vi "RiferimentoTensioneKEB.vi"(11 "Value in":cluster{"Hz":dbl, "V":dbl}) -> (3 "Riferimento Tensione":sgl)   [LabVIEW 2019]
uses:
  Global config keb.vi
  KEB VF status global.vi
panel:
  out "correzione V %":dbl
  in  "%":dbl format="%#_13g"
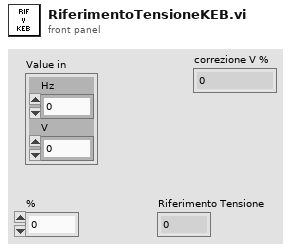
[diagram p1: front panel]
types:
  T1 = typedef "ConfigurazioneKeb.ctl" = cluster{"Freq nom":dbl, "RPM nom":dbl, "Pot nom":dbl, "I nom":dbl, "V nom":dbl, "Rpm max":dbl, "Tipo Motore":dbl}
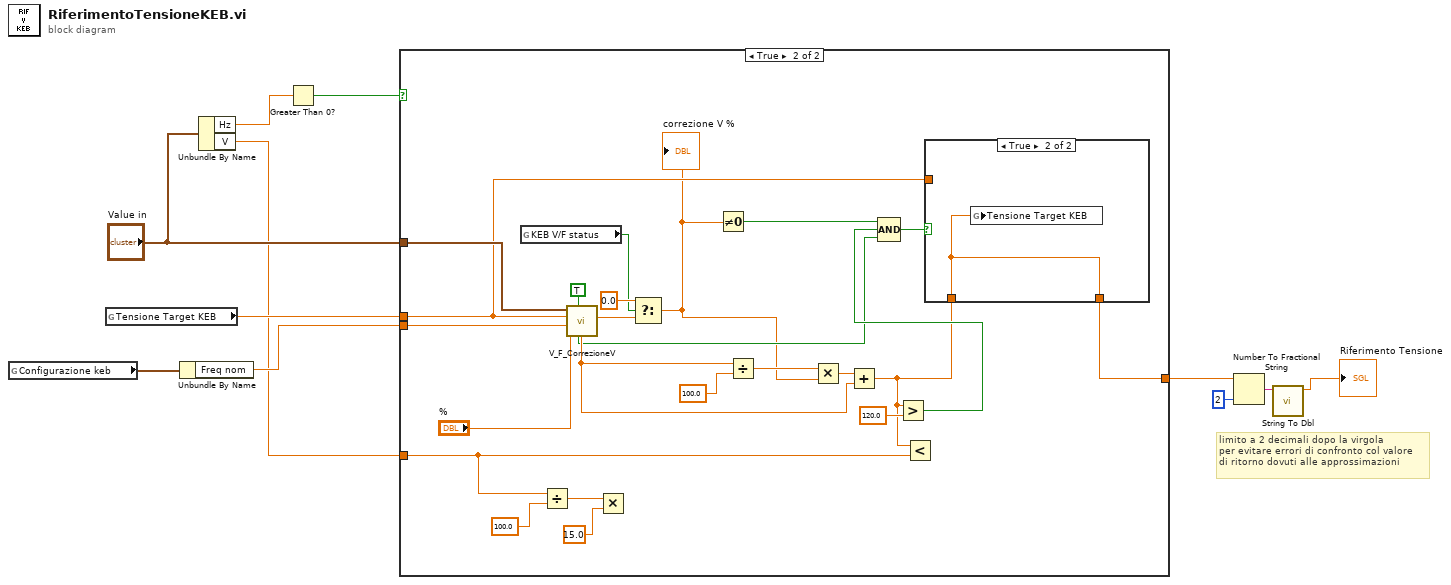
[diagram p0: block diagram]
diagram:
  # "limito a 2 decimali dopo la virgola\nper evitare errori di confronto col valore\ndi ritorno dovuti alle approssimazioni"
  n1 = global read "Global config keb.vi" "Configurazione keb"() -> (w11:T1)
  n2 = global read "Global config keb.vi" "Tensione Target KEB"() -> (w9:dbl)
  n3 = Unbundle By Name(w11) -> ("Freq nom"=w10:dbl)
  n4 = Unbundle By Name("Value in") -> ("Hz"=w7:dbl, "V"=w6:dbl)
  n5 = Greater Than 0?(x=w7) -> (x > 0?=w5:bool)
  n6 = case shown="True" w5 {
    tunnel: w10 -> [_ w33]
    tunnel: "Value in" -> [_ w32]
    tunnel: w9 -> [w12 w23]
    tunnel: [w12 w24] -> w2
    tunnel: w6 -> [_ w17]
    frame False {
    }
    frame True {
      n7 = global read "KEB VF status global.vi" "KEB V/F status"() -> (w13:bool)
      n8 = Divide(x=w17, y=100.0) -> (x/y=w20:dbl)
      n9 = call "V_F_CorrezioneV.vi"("Limita"=TRUE, "%"="%", "Fginocchio"=w33, "Vmax"=w23, "Value in"=w32) -> ("correzione V %"=w16:dbl, "In Range?"=w18:bool)  [unwired: 1 in, 4 out]
      n10 = Multiply(x=w20, y=15.0) -> ()  [unwired: 1 out]
      n11 = Select(t=0.0, s=w13, f=w16) -> (s? t:f=w14:dbl)
      "correzione V %" <- w14
      n12 = Not Equal To 0?(x=w14) -> (x != 0?=w27:bool)
      n13 = Divide(x=w23, y=100.0) -> (x/y=w30:dbl)
      n14 = Multiply(x=w30, y=w14) -> (x*y=w29:dbl)
      n15 = Add(x=w29, y=w23) -> (x+y=w22:dbl)
      n16 = Greater?(x=w22, y=120.0) -> (0:w26:bool)
      n17 = Compound Arithmetic op=AND(w27, w26, w18) -> (w25:bool)
      n18 = Less?(x=w22, y=w17) -> ()  [unwired: 1 out]
      n19 = case shown="True" w25 {
        tunnel: w22 -> [_ w37]
        tunnel: [w36 w37] -> w24
        tunnel: w23 -> [w36 _]
        frame False {
        }
        frame True {
          n20 = global write "Global config keb.vi" "Tensione Target KEB"(w37) -> ()
        }
      }
    }
  }
  n21 = Number To Fractional String(number=w2, precision (6)=i16 2) -> (F-format string=w3:string)  [unwired: 2 in]
  n22 = call "String To Dbl.vi"("String"=w3) -> ("Numeric"=→"Riferimento Tensione":dbl)  [unwired: 10 in]
